vi "DbaseSanityCheck.vi"(8 "error in (no error)":errorcluster, 11 "FAMM in":T1={"FAMM_PAQ_Layers"=0, "FAMM_PAQ_resolution"=0.0, "PAQ_TAGs"=[], "WAQ_TAGs"=[], "EAQ_TAGs"=[], "All_TAGs"=[], "PAQtagProps"=[], "WAQtagProps"=[], "EAQtagProps"=[], "DBAL_class"=refnum, "PAQ_memory"=[], "PAQupdates"=[], "FAMM_Size"={"other"=0, "1day"=0, "1week"=0}, "DatabaseFileExtention"="", "DatabaseSaveRate"=0.0, "Database_path"=path "G:/Sgraph_database", "DBAL-Queue"=refnum, "OS_name"="undefined"} {"FAMM_Size"."1week" format="%.0p"; "FAMM_Size"."1day" format="%.0p"; "FAMM_Size"."other" format="%.0p"; "EAQtagProps"."TagFunc" format="%08x"; "EAQtagProps"."RangeL" format="%.2f"; "EAQtagProps"."RangeH" format="%.2f"; "WAQtagProps"."TagFunc" format="%08x"; "WAQtagProps"."RangeL" format="%.2f"; "WAQtagProps"."RangeH" format="%.2f"; "PAQtagProps"."TagFunc" format="%08x"; "PAQtagProps"."RangeL" format="%.2f"; "PAQtagProps"."RangeH" format="%.2f"; "FAMM_PAQ_resolution" format="%.1p"}) -> (0 "error out":errorcluster, 3 "FAMM out":T1={"FAMM_PAQ_Layers"=0, "FAMM_PAQ_resolution"=0.0, "PAQ_TAGs"=[], "WAQ_TAGs"=[], "EAQ_TAGs"=[], "All_TAGs"=[], "PAQtagProps"=[], "WAQtagProps"=[], "EAQtagProps"=[], "DBAL_class"=refnum, "PAQ_memory"=[], "PAQupdates"=[], "FAMM_Size"={"other"=0, "1day"=0, "1week"=0}, "DatabaseFileExtention"="", "DatabaseSaveRate"=0.0, "Database_path"=path "G:/Sgraph_database", "DBAL-Queue"=refnum, "OS_name"="undefined"} {"FAMM_Size"."1week" format="%.0p"; "FAMM_Size"."1day" format="%.0p"; "FAMM_Size"."other" format="%.0p"; "EAQtagProps"."TagFunc" format="%08x"; "EAQtagProps"."RangeL" format="%.2f"; "EAQtagProps"."RangeH" format="%.2f"; "WAQtagProps"."TagFunc" format="%08x"; "WAQtagProps"."RangeL" format="%.2f"; "WAQtagProps"."RangeH" format="%.2f"; "PAQtagProps"."TagFunc" format="%08x"; "PAQtagProps"."RangeL" format="%.2f"; "PAQtagProps"."RangeH" format="%.2f"; "FAMM_PAQ_resolution" format="%.1p"})   [LabVIEW 2020, in "Sgraph_lib_V1.lvlib" / "FAMM.lvclass"]
doc: "Check if the database exists,\nIf yes and content is OK: then continue.\n\nIf parts are missing: Start user dialog and request what to do."
uses:
  FAMM.lvclass
  controls/FAMM-attributes.ctl
  Common/controls/typedef_com_TagProp.ctl
  DBAL/DBAL.lvclass
  PAQ-memory.lvclass
  DBAL/controls/DBAL_Command.ctl
  DBAL/controls/DBAL-commands.ctl
  Builds/Sgraph_lib_V1.lvlib
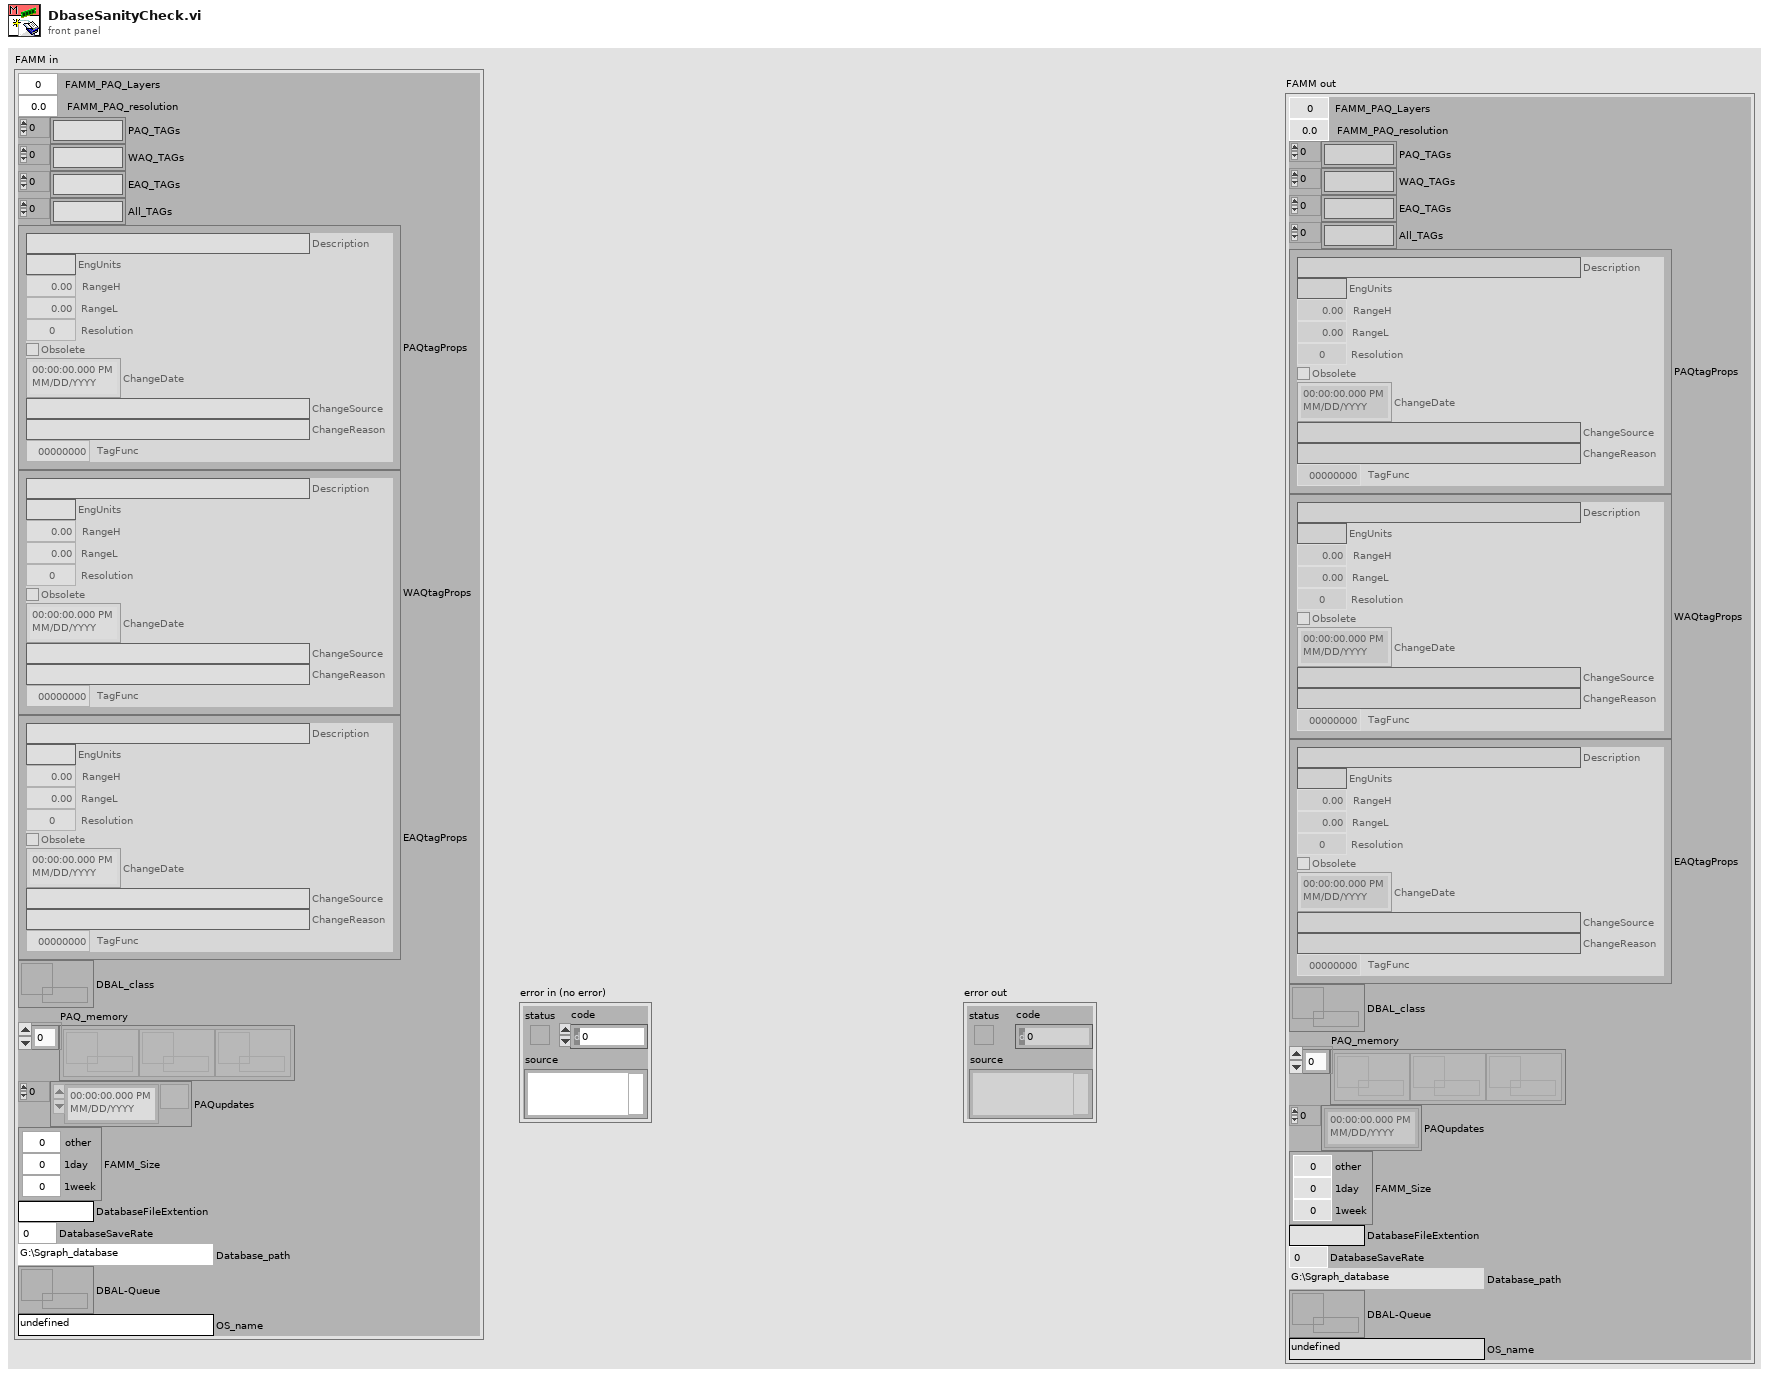
[diagram p1: front panel]
types:
  T1 = typedef "Sgraph_lib_V1.lvlib/FAMM.lvclass/FAMM-attributes.ctl" = cluster{"FAMM_PAQ_Layers":i32, "FAMM_PAQ_resolution":dbl, "PAQ_TAGs":string[], "WAQ_TAGs":string[], "EAQ_TAGs":string[], "All_TAGs":string[], "PAQtagProps":T2[], "WAQtagProps":T2[], "EAQtagProps":T2[], "DBAL_class":refnum<data-value>, "PAQ_memory":refnum<data-value>[], "PAQupdates":timestamp[], "FAMM_Size":cluster{"other":i32, "1day":i32, "1week":i32}, "DatabaseFileExtention":string, "DatabaseSaveRate":dbl, "Database_path":path, "DBAL-Queue":refnum<queue>, "OS_name":string}
  T2 = typedef "Sgraph_lib_V1.lvlib/typedef_com_TagProp.ctl" = cluster{"Description":string, "EngUnits":string, "RangeH":dbl, "RangeL":dbl, "Resolution":i32, "Obsolete":bool, "ChangeDate":timestamp, "ChangeSource":string, "ChangeReason":string, "TagFunc":u32}
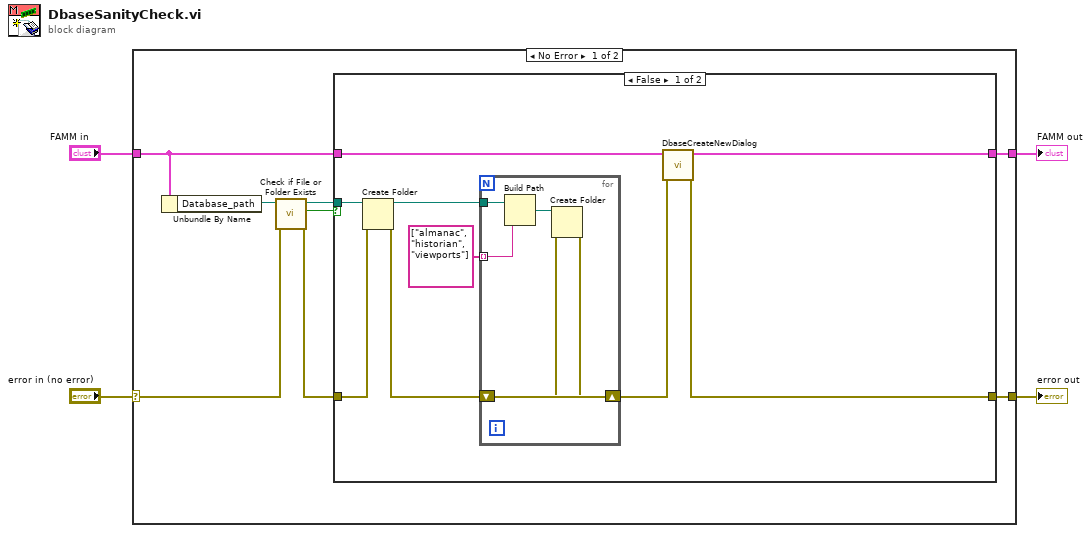
[diagram p0: block diagram]
diagram:
  n1 = case shown="No Error" "error in (no error)" {
    selector: "error in (no error)" -> [w11 w29]
    tunnel: [w6 w29] -> w3
    tunnel: [w8 w28] -> w1
    tunnel: "FAMM in" -> [w9 w28]
    frame No Error {
      n2 = Unbundle By Name(w9) -> ("Database_path"=w12:path)
      n3 = call <vilib>:"Check if File or Folder Exists.vi"("error in (no error)"=w11, "path"=w12) -> ("error out"=w7:errorcluster, "file or folder exists?"=w10:bool, "dup path"=w5:path)  [unwired: 7 in]
      n4 = case shown="False" w10 {
        tunnel: w9 -> [w15 w27]
        tunnel: [w16 w27] -> w8
        tunnel: w7 -> [w19 w26]
        tunnel: [w13 w26] -> w6
        tunnel: w5 -> [w20 _]
        frame False {
          n5 = Create Folder(path (use dialog)=w20, error in=w19) -> (created path=w17:path, error out=w14:errorcluster)  [unwired: 1 in, 1 out]
          n6 = for {
            tunnel: string[] ["almanac", "historian", "viewports"] -> [w24] mode=indexing
            tunnel: w17 -> [w25]
            shift-right: [w21] -> _
            shift-left: w14 -> [w22]
            n7 = Build Path(base path=w25, name or relative path=w24) -> (appended path=w23:path)
            n8 = Create Folder(path (use dialog)=w23, error in=w22) -> (error out=w21:errorcluster)  [unwired: 1 in, 2 out]
          }
          n9 = call "DbaseCreateNewDialog.vi"("error in (no error)"=w14, "FAMM in"=w15) -> ("error out"=w13:errorcluster, "FAMM out"=w16:T1)  [unwired: 8 in]
        }
        frame True {
        }
      }
    }
    frame Error {
    }
  }
  "error out" <- w3
  "FAMM out" <- w1
